vi "cDAQ_MO.vi"(8 "error in":errorcluster) -> (0 "error out":errorcluster, 3 "task out":refnum<k21>)   [LabVIEW 2022 SP3]
uses:
  <vilib>/DAQmx/create/channels.llb/DAQmx Create Channel (AI-Force-Bridge-Two-Point-Linear).vi
  <vilib>/DAQmx/configure/timing.llb/DAQmx Timing (Sample Clock).vi
  <resource>/objmgr/daqmx.rc
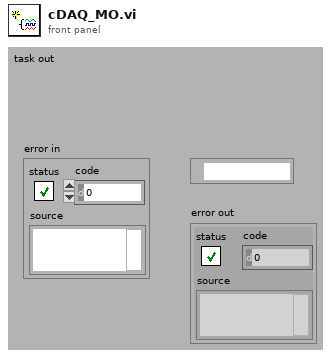
[diagram p1: front panel]
types:
  T1 = cluster{"bridge configuration":i32, "voltage excitation source":i32, "voltage excitation value":dbl, "nominal bridge resistance":dbl}
  T2 = cluster{"first electrical value":dbl, "second electrical value":dbl, "electrical units":i32, "first physical value":dbl, "second physical value":dbl, "physical units":i32}
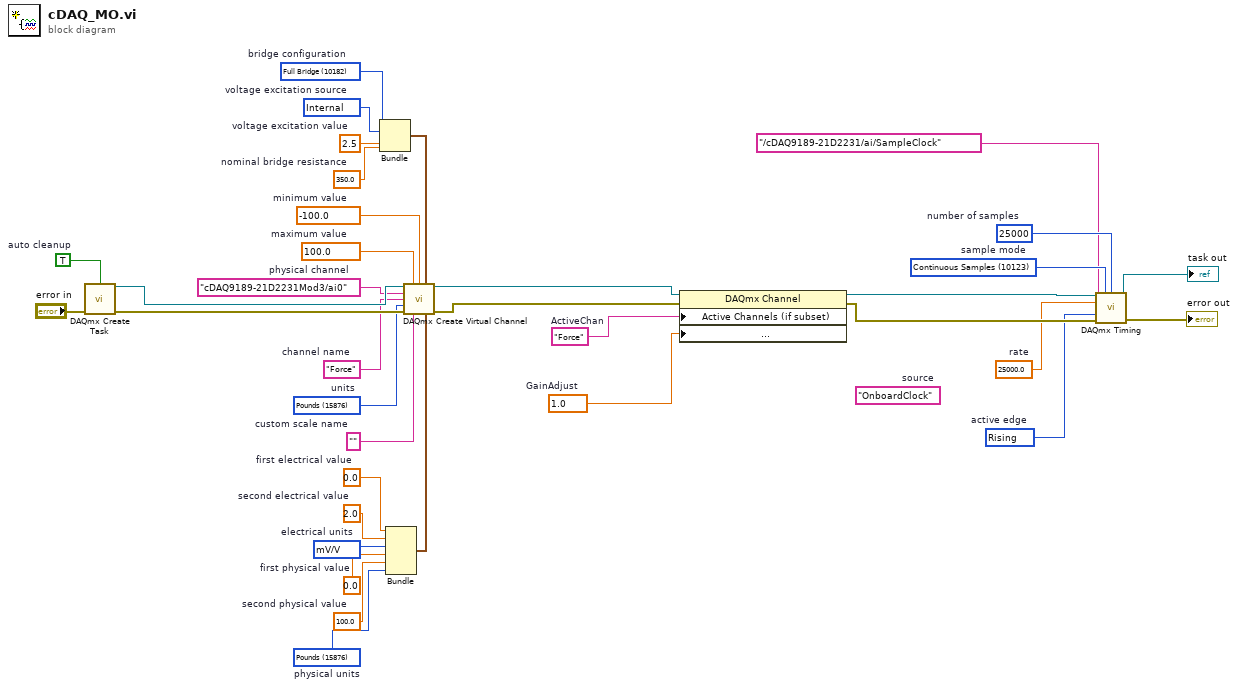
[diagram p0: block diagram]
diagram:
  w2 = 10123 items=["Finite Samples"=10178, "Continuous Samples"=10123, "Hardware Timed Single Point"=12522]  # sample mode
  w3 = 25000.0  # rate
  w4 = 10280 items=["Rising"=10280, "Falling"=10171]  # active edge
  (unwired) "OnboardClock"  # source
  w5 = 25000  # number of samples
  w9 = 1.0  # GainAdjust
  w12 = "Force"  # ActiveChan
  w13 = 15876 items=["Newtons"=15875, "Pounds"=15876, "kgf"=15877]  # physical units
  w19 = 0.0  # first electrical value
  w18 = 2.0  # second electrical value
  w17 = 15897 items=["V/V"=15896, "mV/V"=15897]  # electrical units
  w16 = 0.0  # first physical value
  w15 = 100.0  # second physical value
  w21 = 350.0  # nominal bridge resistance
  w22 = 2.5  # voltage excitation value
  w23 = 10200 items=["Internal"=10200, "External"=10167]  # voltage excitation source
  w24 = 10182 items=["Full Bridge"=10182, "Half Bridge"=10187, "Quarter Bridge"=10270]  # bridge configuration
  w25 = 15876 items=["Newtons"=15875, "Pounds"=15876, "kgf"=15877, "From Custom Scale"=10065]  # units
  w26 = "Force"  # channel name
  w28 = ""  # custom scale name
  w29 = -100.0  # minimum value
  w30 = 100.0  # maximum value
  w31 = "cDAQ9189-21D2231Mod3/ai0"  # physical channel
  w33 = TRUE  # auto cleanup
  n1 = call <vilib>:"DAQmx Create Task.vi"("auto cleanup"=w33, "error in"="error in") -> ("task out"=w32:refnum<k21>, "error out"=w34:errorcluster)  [unwired: 12 in]
  n2 = Bundle("bridge configuration"=w24, "voltage excitation source"=w23, "voltage excitation value"=w22, "nominal bridge resistance"=w21) -> (w20:T1)  [unwired: 1 in]
  n3 = Bundle("first electrical value"=w19, "second electrical value"=w18, "electrical units"=w17, "first physical value"=w16, "second physical value"=w15, "physical units"=w13) -> (w14:T2)  [unwired: 1 in]
  n4 = call-poly <vilib>:"DAQmx Create Virtual Channel.vi"("task in"=w32, "maximum value"=w30, "minimum value"=w29, "bridge information"=w20, "physical channels"=w31, "name to assign"=w26, "units"=w25, "error in"=w34, "custom scale name"=w28, "scaling information"=w14) -> ("task out"=w11:refnum<k21>, "error out"=w27:errorcluster)  [unwired: 4 in]
  n5 = property class="DAQmx Channel"(reference=w11, error in=w27, "Active Channels (if subset)"=w12, "Analog Input:General Properties:Signal Conditioning:Bridge:Shunt Cal:Gain Adjustment"=w9) -> (reference out=w6:refnum<k21>, error out=w10:errorcluster)
  n6 = call-poly <vilib>:"DAQmx Timing.vi"("task/channels in"=w6, "sample mode"=w2, "samples per channel"=w5, "rate"=w3, "source"=tag "/cDAQ9189-21D2231/ai/SampleClock", "active edge"=w4, "error in"=w10) -> ("task out"=→"task out":refnum<k21>, "error out"=→"error out":errorcluster)  [unwired: 7 in]
